vi "Read N channels.vi"(8 "error in (no error)":errorcluster, 11 "device data model in":refnum<class "ET-7042 Data Model.lvclass">) -> (0 "error out":errorcluster, 2 "N channel":T1, 3 "device data model out":refnum<class "ET-7042 Data Model.lvclass">)   [LabVIEW 2021, in "ET-7042 Data Model.lvclass"]
doc: "Retrieves objects from the device model."
uses:
  ET-7042 Data Model.lvclass
  Modbus_v121c/Data Model/N channel.ctl
  ET-7042 Data Model.lvclass/ET-7042 Data Model.ctl
  Modbus_v121c/Data Model/Device Data Model.lvclass
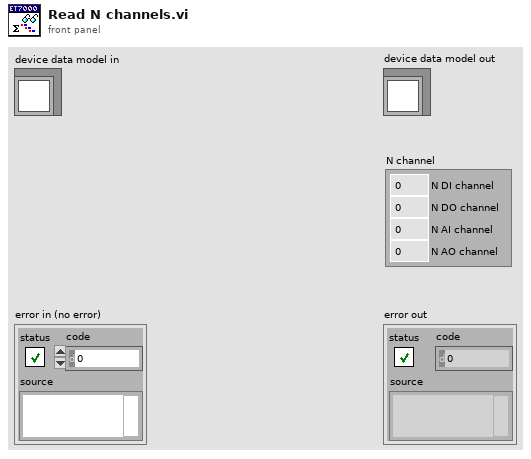
[diagram p1: front panel]
types:
  T1 = typedef "Device Data Model.lvclass/N channel.ctl" = cluster{"N DI channel":i32, "N DO channel":i32, "N AI channel":i32, "N AO channel":i32}
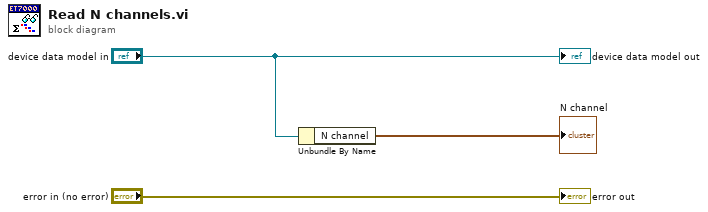
[diagram p0: block diagram]
diagram:
  n1 = Unbundle By Name("device data model in") -> ("N channel"=→"N channel":T1)
  "error out" <- "error in (no error)"
  "device data model out" <- "device data model in"
